vi "CLD 15 Text String Parsing Front Panel.vi"(8 "Error In":errorcluster) -> (0 "Error Out":errorcluster)   [LabVIEW 2009]
doc: "CLD 15 exercise"
uses:
  CLD 15 CSV file data structure.ctl
panel:
  out "File Data":string[][](array[string])
  out "Data Saved to File":string[][](array[string])
  out "processed Data":T1[](array[typedef])
  # "Processed Data"
  # "Input Data"
  # "Output Data"
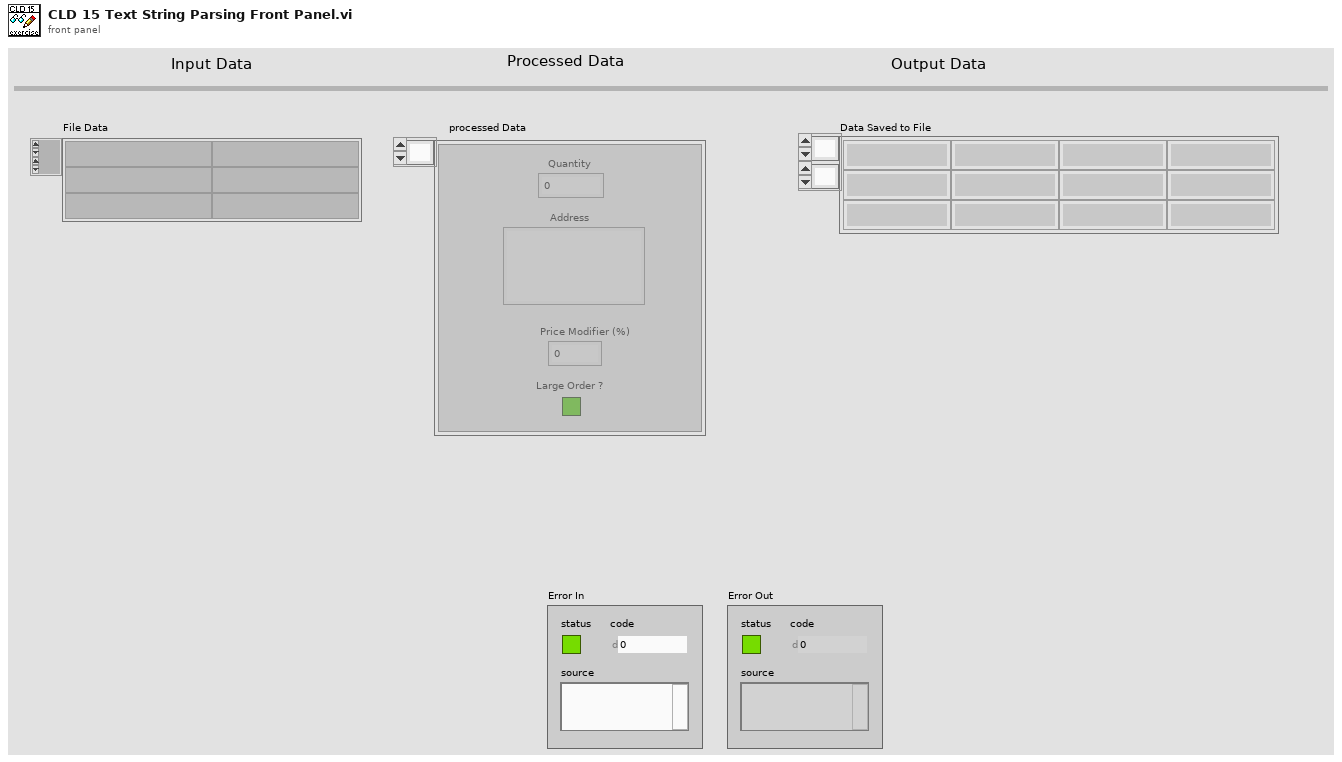
[diagram p1: front panel]
types:
  T1 = typedef "CLD 15 CSV file data structure.ctl" = cluster{"Quantity":i32, "Address":string, "Price Modifier (%)":dbl, "Large Order ?":bool}
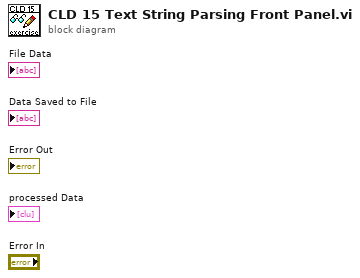
[diagram p0: block diagram]
diagram:
